vi "Set Timer.vi"(8 "error in (no error)":errorcluster, 9 "User":bool, 10 "Admin":bool, 11 "Master in":refnum<class "Master.lvclass">) -> (0 "error out":errorcluster, 1 "Done":bool, 2 "Cluster":cluster{"minute":i32, "hour":i32}, 3 "Master out":refnum<class "Master.lvclass">, 4 "Running":bool, 5 "Time":dbl)   [LabVIEW 2014, in "Master.lvclass"]
uses:
  Master/Master.lvclass
  Controls/StateTimer.ctl
  Master/Master.lvclass/Master.ctl
  Controls/Control Library.lvlib
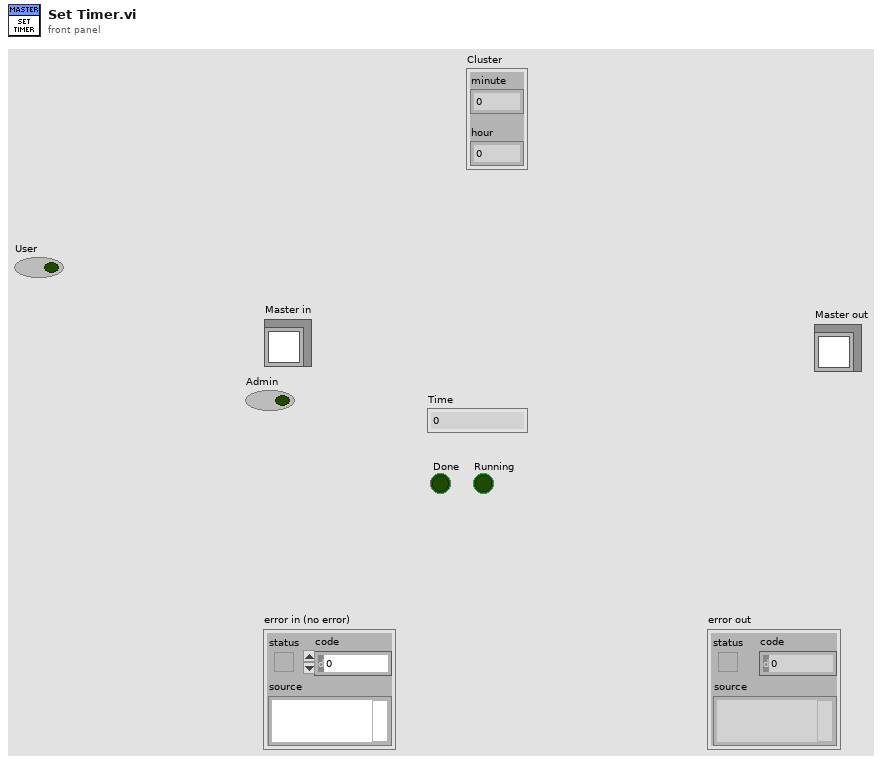
[diagram p1: front panel]
types:
  T1 = typedef "Control Library.lvlib/StateTimer.ctl" = enum16{"Initialize", "RealTime", "Pause", "Stop"}
  T2 = typedef "LVDateTimeRec.ctl" = cluster{"fractional second":dbl, "second":i32, "minute":i32, "hour":i32, "day of month":i32, "month":i32, "year":i32, "day of week":i32, "day of year":i32, "DST":i32}
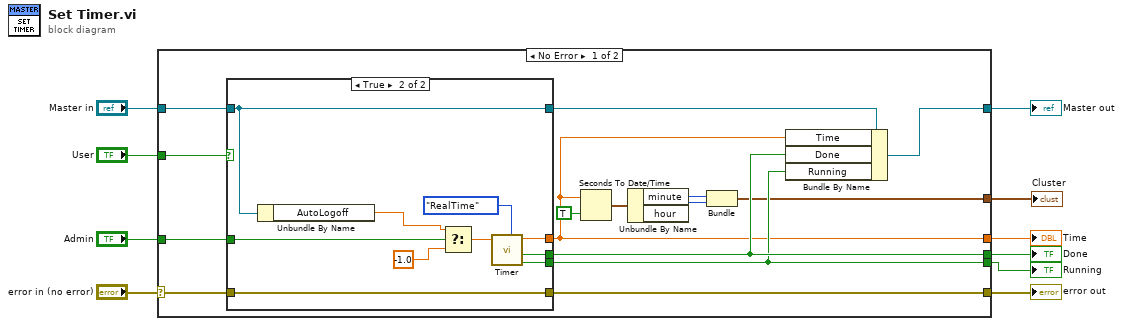
[diagram p0: block diagram]
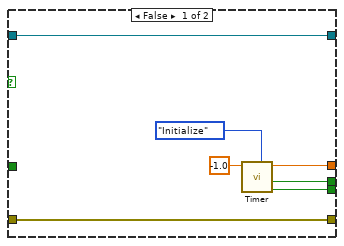
[diagram p2: hidden frame]
diagram:
  n1 = case shown="No Error" "error in (no error)" {
    selector: "error in (no error)" -> [w24 w44]
    tunnel: [w15 w44] -> w9
    tunnel: [w23 w43] -> w7
    tunnel: "Master in" -> [w25 w43]
    tunnel: "Admin" -> [w13 _]
    tunnel: [w12 _] -> w5
    tunnel: [w22 _] -> w4
    tunnel: [w21 _] -> w3
    tunnel: "User" -> [w14 _]
    tunnel: [w17 _] -> w1
    frame No Error {
      n2 = case shown="True" w14 {
        tunnel: [w32 w34] -> w16
        tunnel: w25 -> [w32 w34]
        tunnel: w24 -> [w31 w42]
        tunnel: [w31 w42] -> w15
        tunnel: [w28 w40] -> w12
        tunnel: [w27 w39] -> w22
        tunnel: [w26 w38] -> w21
        tunnel: w13 -> [_ w37]
        frame False {
          n3 = call "Timer.vi"("StateTimer"=StateTimer."Initialize", "Setpoint"=-1.0 ("Setpoint Timer")) -> ("Running"=w26:bool, "Done"=w27:bool, "Time"=w28:dbl)  [unwired: 7 in]
        }
        frame True {
          n4 = Unbundle By Name(w34) -> ("AutoLogoff"=w33:dbl)
          n5 = Select(t=w33, s=w37, f=-1.0) -> (s? t:f=w36:dbl)
          n6 = call "Timer.vi"("StateTimer"=StateTimer."RealTime", "Setpoint"=w36) -> ("Running"=w38:bool, "Done"=w39:bool, "Time"=w40:dbl)  [unwired: 7 in]
        }
      }
      n7 = Seconds To Date/Time(time stamp (now)=w12, to UTC (F)=TRUE) -> (date time rec=w20:T2)
      n8 = Unbundle By Name(w20) -> ("minute"=w19:i32, "hour"=w18:i32)
      n9 = Bundle("minute"=w19, "hour"=w18) -> (w17:cluster{"minute":i32, "hour":i32})  [unwired: 1 in]
      n10 = Bundle By Name(cluster=w16, "Time"=w12, "Done"=w22, "Running"=w21) -> (w23:refnum<class "Master.lvclass">)
    }
    frame Error {
    }
  }
  "error out" <- w9
  "Master out" <- w7
  "Done" <- w4
  "Time" <- w5
  "Running" <- w3
  "Cluster" <- w1
